vi "Find Valid Item Ref.vi"(8 "error in (no error)":errorcluster, 9 "scalar channels":T2 {"Data Type" format="%.0x"}, 10 "bitfile object names":string[](array[string]), 11 "section children refs":T1[](array[typedef]) format="%.0x") -> (0 "error out":errorcluster, 1 "scalar channel out":T2 {"Data Type" format="%.0x"}, 2 "found":bool, 3 "item ref out":T1 format="%.0x")   [LabVIEW 2018, in "FPGA Addon System Explorer.lvlib"]
uses:
  FPGA Addon System Explorer.lvlib
  Addon Shared/Types/Register Information.ctl
  Addon Shared/Types/FPGA Addon Data Type.ctl
  <vilib>/NI Veristand/Custom Device API/Custom Device Item Ref.ctl
  <vilib>/NI Veristand/Custom Device API/Custom Device API.lvlib
  Addon Shared/FPGA Addon Shared.lvlib
panel:
  out "section children refs out":T1[](array[typedef]) format="%.0x"
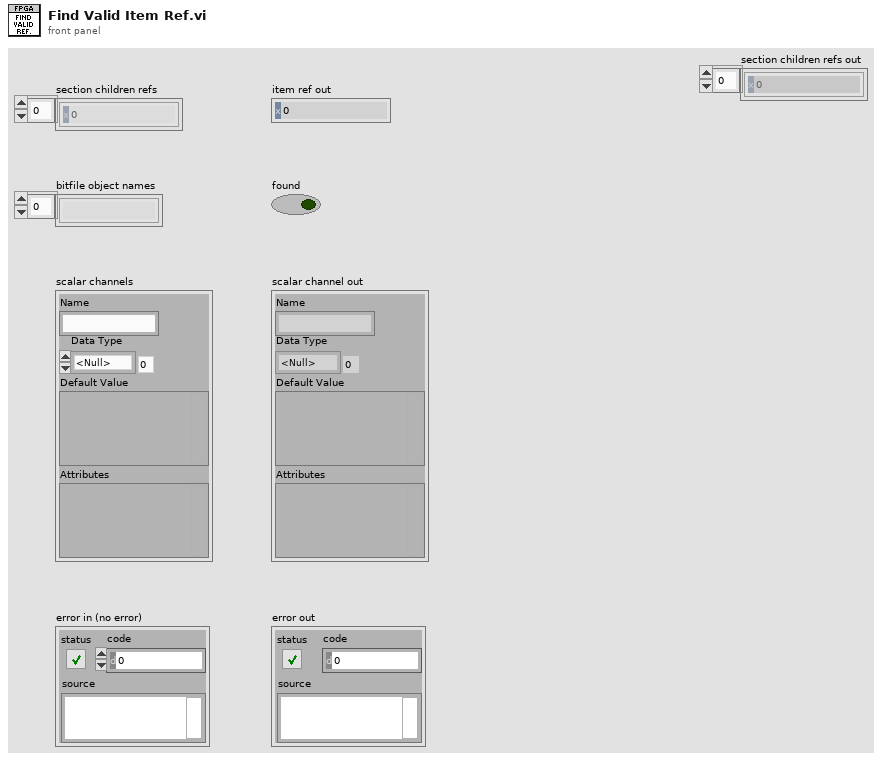
[diagram p1: front panel]
types:
  T1 = typedef "Custom Device API.lvlib/Custom Device Item Ref.ctl" = u64
  T2 = typedef "FPGA Addon Shared.lvlib/Register Information.ctl" = cluster{"Name":string, "Data Type":T3, "Default Value":variant, "Attributes":variant}
  T3 = typedef "FPGA Addon Shared.lvlib/FPGA Addon Data Type.ctl" = enum8{"<Null>", "I8", "I16", "I32", "I64", "U8", "U16", "U32", "U64", "SGL", "Boolean", "Analog PWM In Settings", "Analog PWM In", "Digital PWM In Settings", "Digital PWM In", "Digital PWM Out", "Sine Out", "FXP", "FXP+/-24.5", "FXP+/-16.5", "FXP+/-32.8", "FXP+/-64.32", "FXP+/-16.7", "FXP+/-20.5", "FXP+/-27.5", "FXP+/-32.16", "FXP+16.3", "FXP+18.3", "Digital Static In", "Digital Static Out", "Digital Static In Settings", "Digital WSS Out", "Quad Encoder Settings", "Quad Encoder In", "Group"}
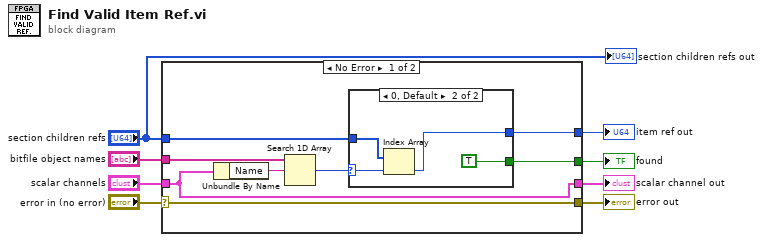
[diagram p0: block diagram]
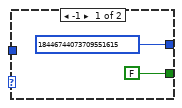
[diagram p2: hidden frame]
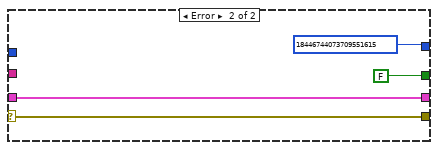
[diagram p3: hidden frame]
diagram:
  n1 = case shown="No Error" "error in (no error)" {
    selector: "error in (no error)" -> [w9 w26]
    tunnel: [w11 w23] -> w8
    tunnel: [w13 T1 18446744073709551615 ("Scalar Section ref")] -> w7
    tunnel: [w12 FALSE ("Not a Ref")] -> w6
    tunnel: [w9 w26] -> w5
    tunnel: "section children refs" -> [w14 _]
    tunnel: "scalar channels" -> [w11 w23]
    tunnel: "bitfile object names" -> [w10 _]
    frame No Error {
      n2 = Unbundle By Name(w11) -> ("Name"=w16:string)
      n3 = Search 1D Array(1D array=w10, element=w16) -> (index of element=w15:i32)  [unwired: 1 in]
      n4 = case shown="0, Default" w15 {
        selector: w15 -> [_ w21]
        tunnel: w14 -> [_ w22]
        tunnel: [T1 18446744073709551615 ("Scalar Section ref") w20] -> w13
        tunnel: [FALSE TRUE] -> w12
        frame -1 {
        }
        frame 0, Default {
          n5 = Index Array(array=w22, index=w21) -> (element=w20:T1)
        }
      }
    }
    frame Error {
    }
  }
  "scalar channel out" <- w8
  "item ref out" <- w7
  "found" <- w6
  "error out" <- w5
  "section children refs out" <- "section children refs"
